vi "Advanced Features.vi"() -> ()   [LabVIEW 2016]
doc: "This example shows advanced features such as limits, units and calibration.\n\nHardware setup: At least one Fluigent pressure controller (MFCS, MFCS-EZ or FlowEZ) and/or one Fluigent sensor (flow-unit connected to FRP or FlowEZ)"
uses:
  fgt_SDK.lvlib
  TypeDefs/fgt_PRESSURE_UNIT.ctl
  TypeDefs/fgt_SENSOR_UNIT.ctl
  TypeDefs/fgt_SENSOR_CALIBRATION.ctl
panel:
  in  "Init":bool=TRUE
  in  "Stop":bool
  in  "Tab Control":T1(tab)
  in  "Apply unit change":bool
  out "Pressure initial value":dbl format="%#_3g"
  out "Sensor's initial value":dbl format="%#_3g"
  out "Sensor's final value":dbl format="%#_3g"
  out "Pressure final value":dbl format="%#_3g"
  in  "New pressure unit":T2
  in  "New flowrate unit":T3
  out "Pressure initial unit":T2
  out "Sensor's initial unit":T3
  out "Sensor's final unit":T3
  out "Pressure final unit":T2
  out "unit out 2":T2
  in  "Set pressure":bool
  in  "Pressure":sgl
  in  "Set limit":bool
  in  "Pmin":sgl
  in  "Pmax":sgl=1.0
  out "unit out":T2
  out "Error string":string
  in  "Calibrate":bool
  in  "Set pressure 2":bool
  in  "Pressure":sgl
  in  "Calibrate sensor":bool
  in  "Read sensor calibration":bool
  out "Current calibration":T4=enum."H2O"
  in  "New calibration table":T4=enum."H2O"
  out "error out":errorcluster
  # "Hit the \"Run\" button, and browse though tabs."
  # "1. Set pressure limits"
  # "2. Try setting pressure over the configured limit"
  # "1. Calibrate the instrument"
  # "2. Try setting the pressure right after having calibrated the instrument"
  # "1. Read sensor's calibration table"
  # "1. Set sensor's calibration table"
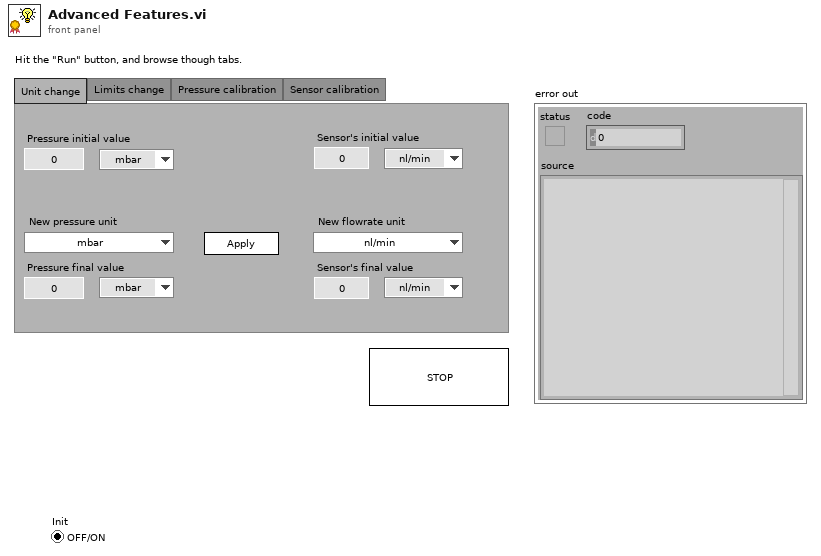
[diagram p1: front panel]
types:
  T1 = enum32{"Unit change", "Limits change", "Pressure calibration", "Sensor calibration"}
  T2 = typedef "fgt_SDK.lvlib/fgt_PRESSURE_UNIT.ctl" = enum16{"mbar", "kPa", "PSI"}
  T3 = typedef "fgt_SDK.lvlib/fgt_SENSOR_UNIT.ctl" = enum16{"nl/min", "µl/s", "µl/min", "ul/h", "ml/min", "ml/h", "mbar", "kPa", "bar"}
  T4 = typedef "fgt_SDK.lvlib/fgt_SENSOR_CALIBRATION.ctl" = enum16{"None", "H2O", "IPA", "HFE", "FC40", "OIL"}
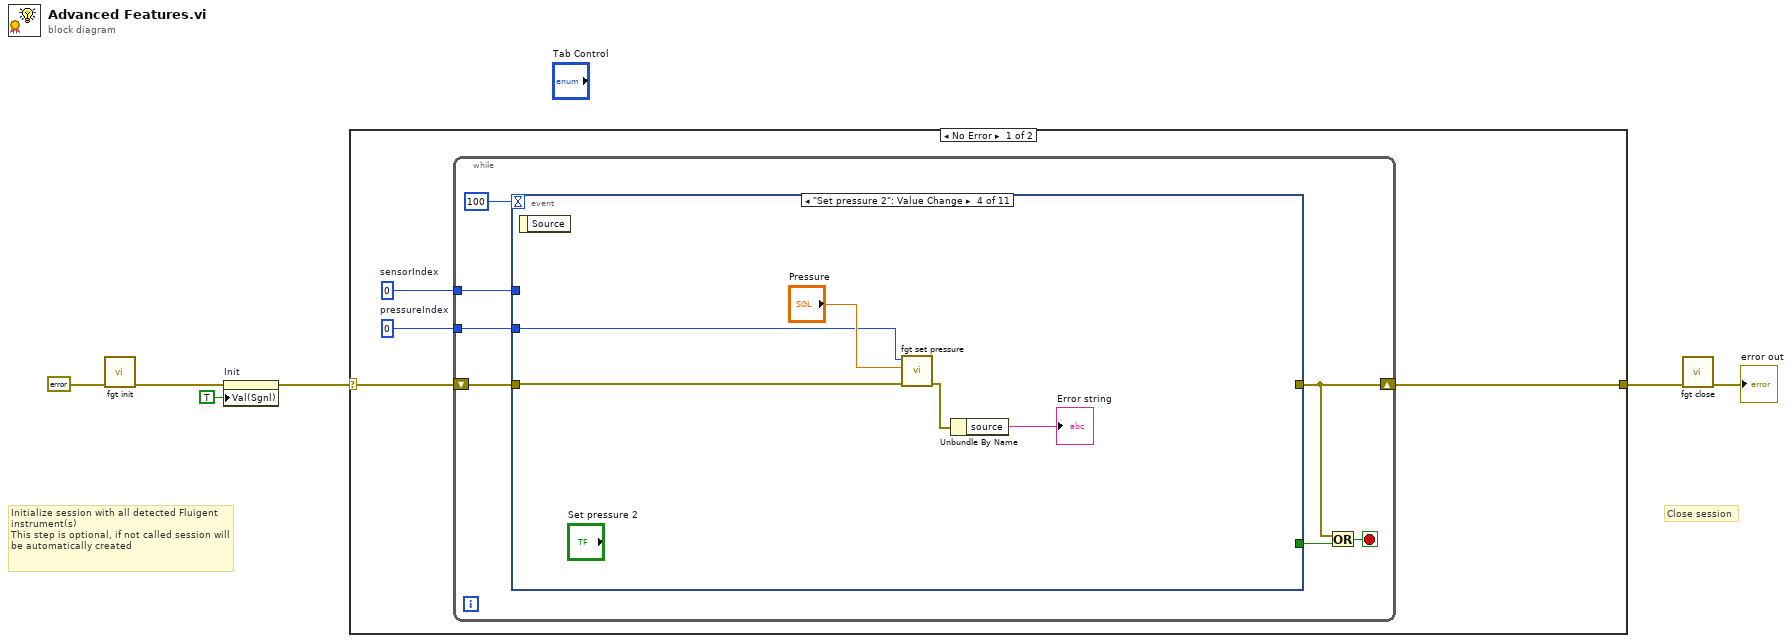
[diagram p0: block diagram]
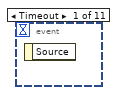
[diagram p2: hidden frame]
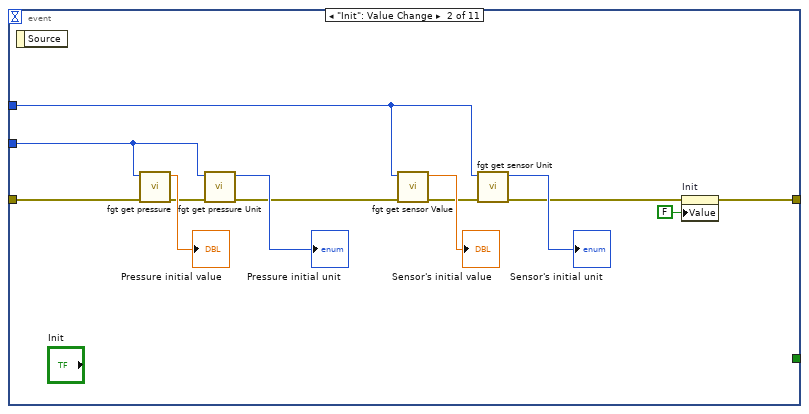
[diagram p3: hidden frame]
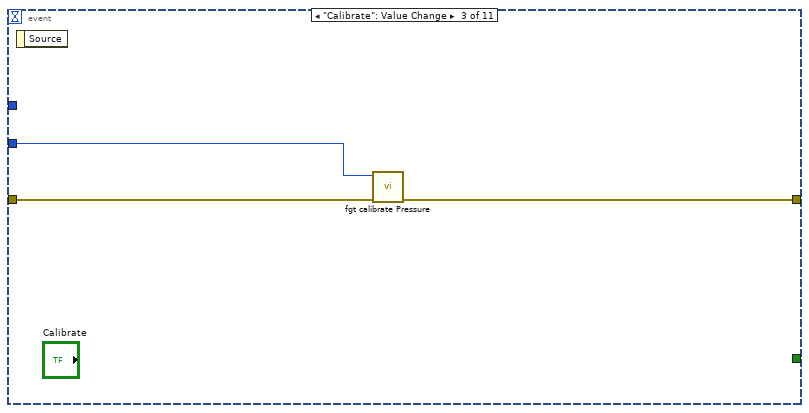
[diagram p4: hidden frame]
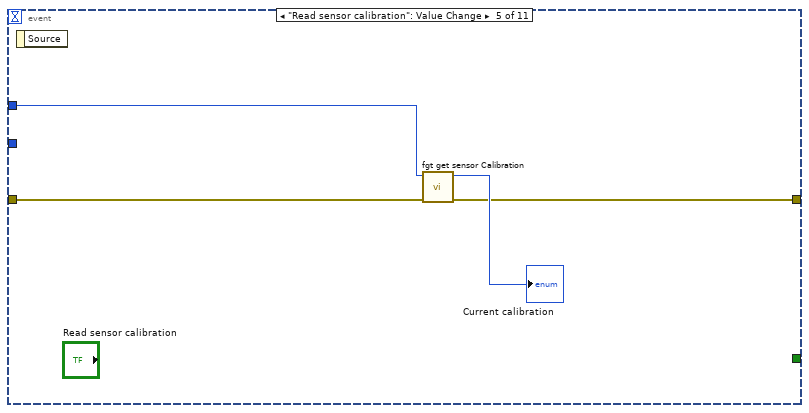
[diagram p5: hidden frame]
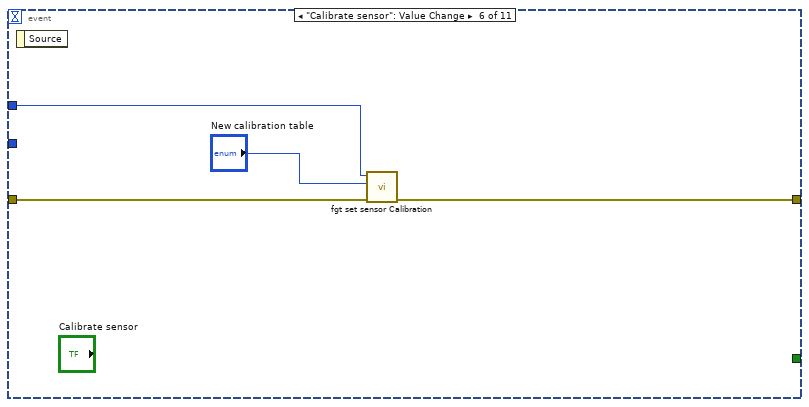
[diagram p6: hidden frame]
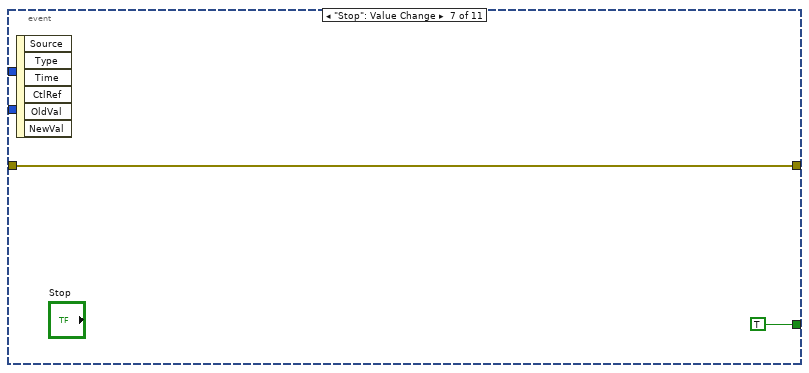
[diagram p7: hidden frame]
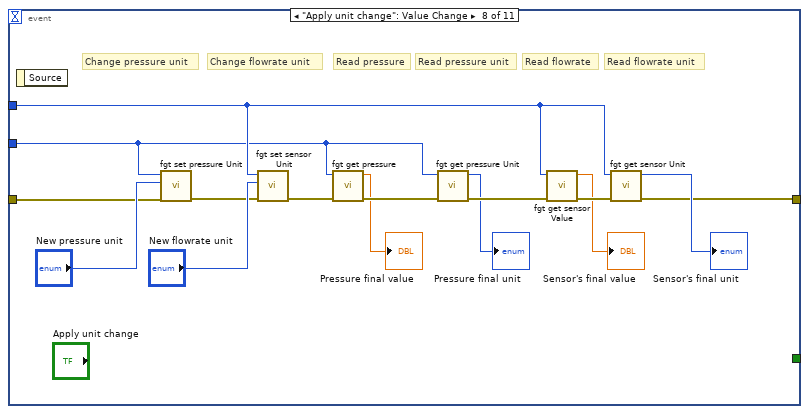
[diagram p8: hidden frame]
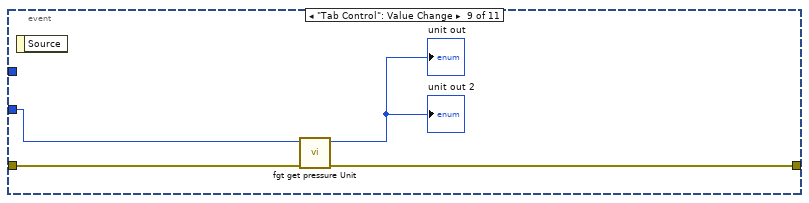
[diagram p9: hidden frame]
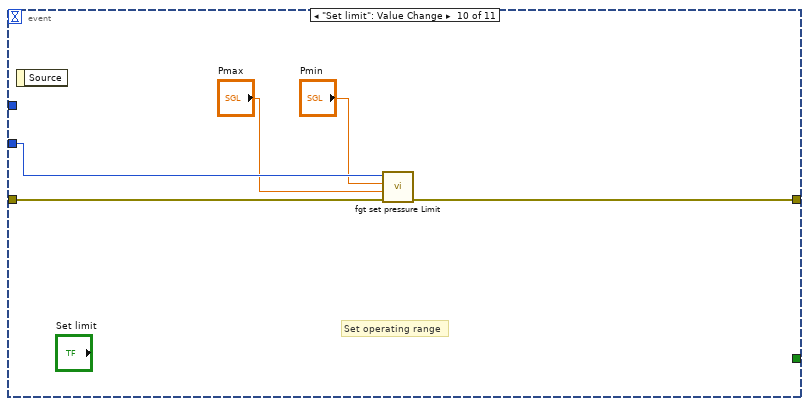
[diagram p10: hidden frame]
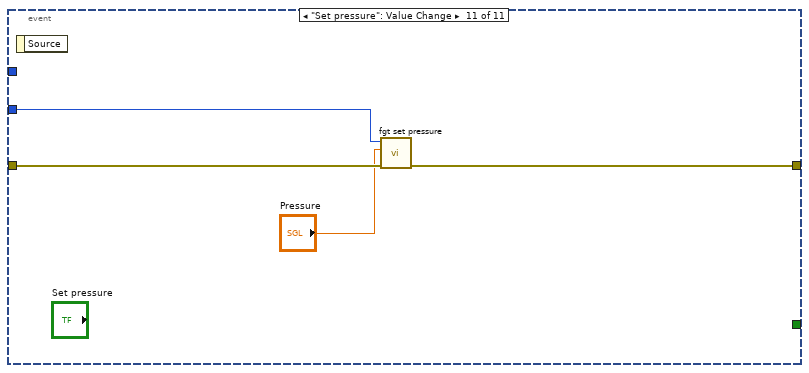
[diagram p11: hidden frame]
diagram:
  # "Close session"
  # "Initialize session with all detected Fluigent instrument(s)\nThis step is optional, if not called session will be automatically created"
  n1 = call "fgt init.vi"("error in (no error)"=errorcluster {"status"=FALSE, "code"=0, "source"=""}) -> ("error out"=w3:errorcluster)  [unwired: 10 in]
  n2 = property on="Init" class="Bool (strict)"(error in=w3, "Val(Sgnl)"=TRUE ("Value (Signaling)")) -> (error out=w2:errorcluster)  [unwired: 1 in, 1 out]
  n3 = case shown="No Error" w2 {
    selector: w2 -> [w9 w77]
    tunnel: [w10 w77] -> w5
    frame No Error {
      w8 = u32 0  # sensorIndex
      w7 = u32 0  # pressureIndex
      n4 = while {
        shift-right: [w11] -> w10
        shift-left: w9 -> [w16]
        tunnel: w8 -> [w14]
        tunnel: w7 -> [w13]
        stop <- w12 stop-if-true
        n5 = event shown="[3] \"Set pressure 2\": Value Change" {
          selector: _ -> [_ _ _ _ _ _ _ _ _ _ _]
          dyn-events: _ -> [_ _ _ _ _ _ _ _ _ _ _]
          timeout: 100 -> [_ _ _ _ _ _ _ _ _ _ _]
          tunnel: [_ _ _ _ _ _ TRUE _ _ _ _] -> w17
          tunnel: [_ w18 w31 _ w39 w43 w47 w51 w65 w68 w73] -> w11
          tunnel: w16 -> [_ w23 w32 w36 w42 w46 w47 w60 w66 w72 w76]
          tunnel: w14 -> [_ w22 _ _ w41 w45 _ w50 _ _ _]
          tunnel: w13 -> [_ w21 w33 w37 _ _ _ w49 w67 w71 w75]
          event Timeout {
            n6 = event-data() -> ()  [unwired: 1 in, 1 out]
          }
          event "Init": Value Change {
            n7 = event-data() -> ()  [unwired: 1 in, 1 out]
            n8 = call "fgt get pressure.vi"("error in (no error)"=w23, "pressureIndex"=w21) -> ("error out"=w24:errorcluster, "pressure out"=→"Pressure initial value":sgl)  [unwired: 8 in]
            n9 = call "fgt get pressure Unit.vi"("error in (no error)"=w24, "pressureIndex"=w21) -> ("error out"=w25:errorcluster, "unit out"=→"Pressure initial unit":T2)  [unwired: 8 in]
            n10 = call "fgt get sensor Value.vi"("error in (no error)"=w25, "sensorIndex"=w22) -> ("error out"=w26:errorcluster, "value out"=→"Sensor's initial value":sgl)  [unwired: 8 in]
            n11 = call "fgt get sensor Unit.vi"("error in (no error)"=w26, "sensorIndex"=w22) -> ("error out"=w19:errorcluster, "unit out"=→"Sensor's initial unit":T3)  [unwired: 8 in]
            n12 = property on="Init" class="Bool (strict)"(error in=w19, "Value"=FALSE ("Init")) -> (error out=w18:errorcluster)  [unwired: 1 in, 1 out]
          }
          event "Calibrate": Value Change {
            n13 = event-data() -> ()  [unwired: 1 in, 1 out]
            n14 = call "fgt calibrate Pressure.vi"("error in (no error)"=w32, "pressureIndex"=w33) -> ("error out"=w31:errorcluster)  [unwired: 9 in]
          }
          event "Set pressure 2": Value Change {
            n15 = event-data() -> ()  [unwired: 1 in, 1 out]
            n16 = call "fgt set pressure.vi"("error in (no error)"=w36, "pressure"="Pressure", "pressureIndex"=w37) -> ("error out"=w35:errorcluster)  [unwired: 8 in]
            n17 = Unbundle By Name(w35) -> ("source"=→"Error string":string)
          }
          event "Read sensor calibration": Value Change {
            n18 = event-data() -> ()  [unwired: 1 in, 1 out]
            n19 = call "fgt get sensor Calibration.vi"("error in (no error)"=w42, "sensorIndex"=w41) -> ("error out"=w39:errorcluster, "calibration out"=→"Current calibration":T4)  [unwired: 8 in]
          }
          event "Calibrate sensor": Value Change {
            n20 = event-data() -> ()  [unwired: 1 in, 1 out]
            n21 = call "fgt set sensor Calibration.vi"("error in (no error)"=w46, "calibration"="New calibration table", "sensorIndex"=w45) -> ("error out"=w43:errorcluster)  [unwired: 8 in]
          }
          event "Stop": Value Change {
            n22 = event-data() -> ()  [unwired: 1 in, 6 out]
          }
          event "Apply unit change": Value Change {
            # "Read flowrate unit"
            # "Read flowrate"
            # "Read pressure unit"
            # "Read pressure"
            # "Change flowrate unit"
            # "Change pressure unit"
            n23 = event-data() -> ()  [unwired: 1 in, 1 out]
            n24 = call "fgt set pressure Unit.vi"("error in (no error)"=w60, "unit"="New pressure unit", "presureIndex"=w49) -> ("error out"=w61:errorcluster)  [unwired: 8 in]
            n25 = call "fgt set sensor Unit.vi"("error in (no error)"=w61, "unit"="New flowrate unit", "sensorIndex"=w50) -> ("error out"=w52:errorcluster)  [unwired: 8 in]
            n26 = call "fgt get pressure.vi"("error in (no error)"=w52, "pressureIndex"=w49) -> ("error out"=w57:errorcluster, "pressure out"=→"Pressure final value":sgl)  [unwired: 8 in]
            n27 = call "fgt get pressure Unit.vi"("error in (no error)"=w57, "pressureIndex"=w49) -> ("error out"=w58:errorcluster, "unit out"=→"Pressure final unit":T2)  [unwired: 8 in]
            n28 = call "fgt get sensor Value.vi"("error in (no error)"=w58, "sensorIndex"=w50) -> ("error out"=w59:errorcluster, "value out"=→"Sensor's final value":sgl)  [unwired: 8 in]
            n29 = call "fgt get sensor Unit.vi"("error in (no error)"=w59, "sensorIndex"=w50) -> ("error out"=w51:errorcluster, "unit out"=→"Sensor's final unit":T3)  [unwired: 8 in]
          }
          event "Tab Control": Value Change {
            n30 = event-data() -> ()  [unwired: 1 in, 1 out]
            n31 = call "fgt get pressure Unit.vi"("error in (no error)"=w66, "pressureIndex"=w67) -> ("error out"=w65:errorcluster, "unit out"=→"unit out" →"unit out 2":T2)  [unwired: 8 in]
          }
          event "Set limit": Value Change {
            # "Set operating range"
            n32 = event-data() -> ()  [unwired: 1 in, 1 out]
            n33 = call "fgt set pressure Limit.vi"("error in (no error)"=w72, "PlimMax"="Pmax", "PlimMin"="Pmin", "pressureIndex"=w71) -> ("error out"=w68:errorcluster)  [unwired: 7 in]
          }
          event "Set pressure": Value Change {
            n34 = event-data() -> ()  [unwired: 1 in, 1 out]
            n35 = call "fgt set pressure.vi"("error in (no error)"=w76, "pressure"="Pressure", "pressureIndex"=w75) -> ("error out"=w73:errorcluster)  [unwired: 8 in]
          }
        }
        n36 = Or(x=w11, y=w17) -> (x .or. y?=w12:bool)
      }
    }
    frame Error {
    }
  }
  n37 = call "fgt close.vi"("error in (no error)"=w5) -> ("error out"=→"error out":errorcluster)  [unwired: 10 in]
